vi "stiffbackReference.vi"() -> ()   [LabVIEW 2015]
uses:
  GlobalPath.vi
  GlobalData.vi
panel:
  in  "DONE ALL?":bool
  out "Mapping file Ext dx":string
  out "Mapping file Ext sx":string
  out "Mapping file Int dx":string
  out "Mapping file Int sx":string
  out "appended path":path
  out "Mapping file pillar":string
  in  "Open Program 5":bool
  out "PanelName":string
  in  "Done with reference plate mapping?":bool
  in  "Open Program":bool
  # "1. Stiffback plate mapping"
  # "At this point, the PCB on the table/stiffback will be tested in the appropriate vi program"
  # "PCB MAPPING"
  # "FRAME/COOLING BAR MAPPING"
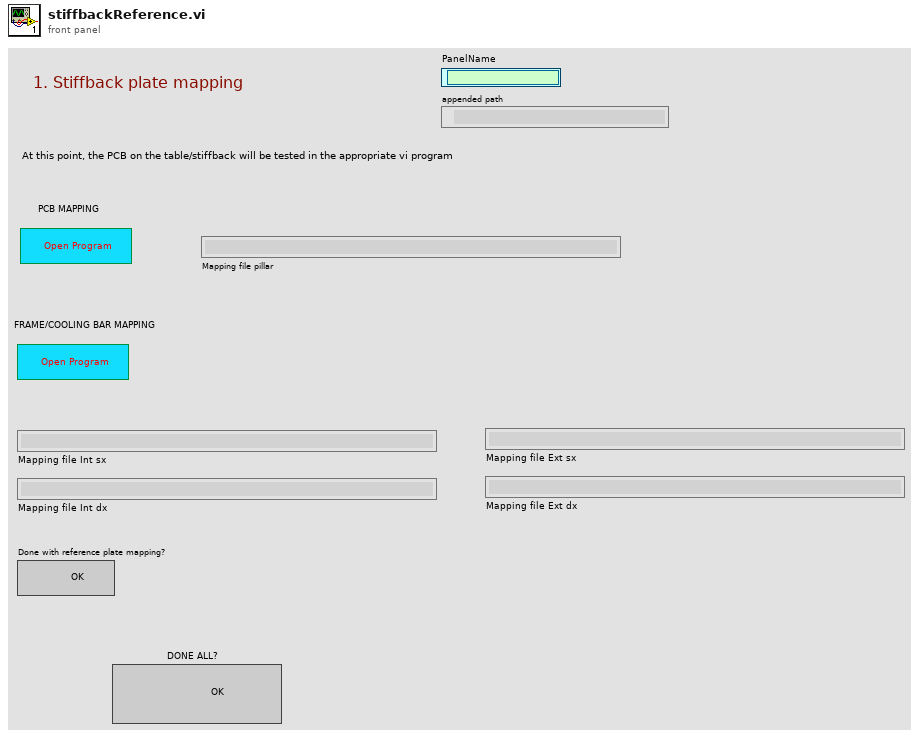
[diagram p1: front panel]
types:
  T1 = enum16{"open", "replace", "create", "open or create", "replace or create", "replace or create with confirmation"}
  T2 = enum32{"Bad", "Idle", "Run top level", "Running"}
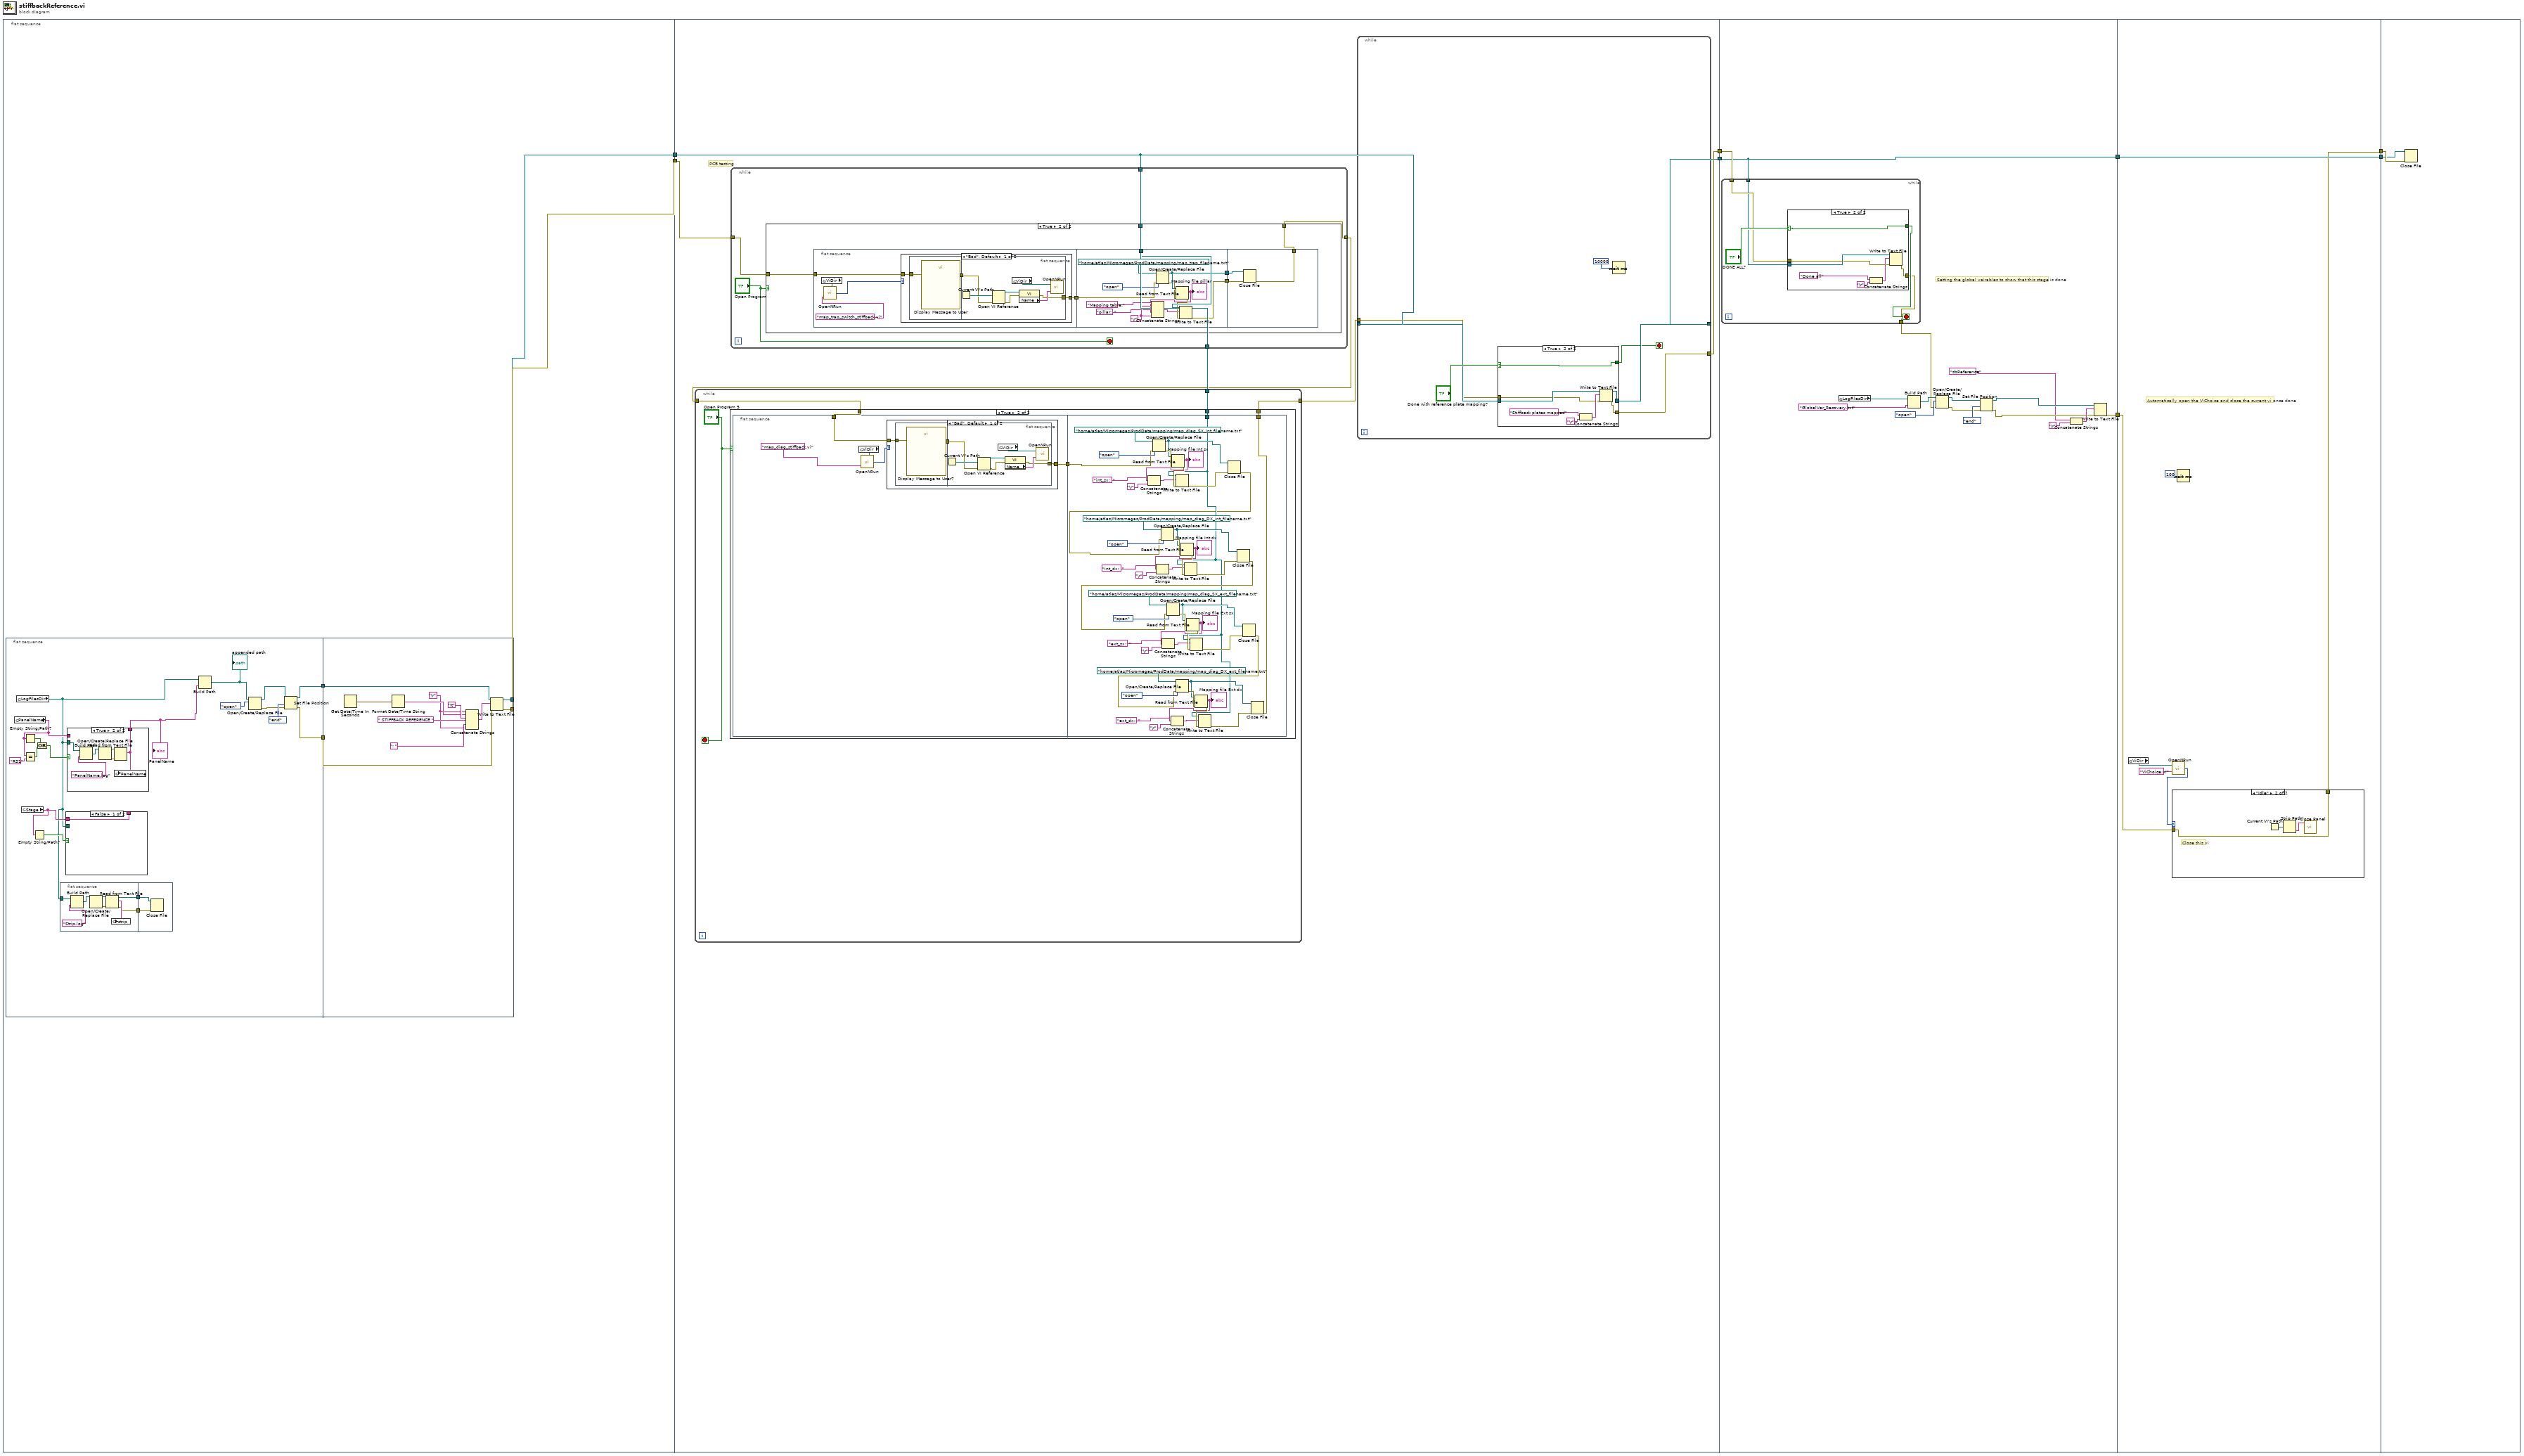
[diagram p0: block diagram]
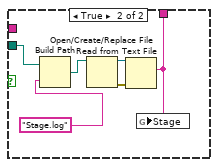
[diagram p2: hidden frame]
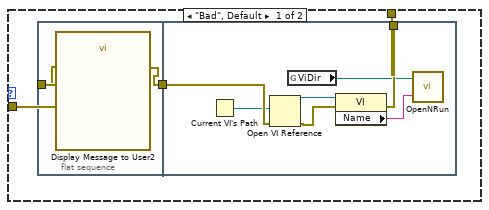
[diagram p10: hidden frame]
diagram:
  n1 = flat-sequence {
    tunnel: [w11] -> w2
    tunnel: [w9] -> w1
    tunnel: w2 -> [w72]
    tunnel: [w66] -> w8
    tunnel: [w71] -> w7
    tunnel: w1 -> [w67]
    tunnel: w8 -> [w212]
    tunnel: w7 -> [w210]
    tunnel: [w210] -> w6
    tunnel: [w214] -> w4
    tunnel: w6 -> [w245]
    tunnel: [w245] -> w5
    tunnel: w4 -> [w241]
    tunnel: [w240] -> w3
    tunnel: w5 -> [w261]
    tunnel: w3 -> [w262]
    frame #0 {
      n2 = flat-sequence {
        tunnel: [w25] -> w12
        tunnel: [w24] -> w10
        tunnel: w12 -> [w61]
        tunnel: [w60] -> w9
        tunnel: [w59] -> w11
        tunnel: w10 -> [w58]
        frame #0 {
          n3 = global read "GlobalData.vi" "PanelName"() -> (w18:string)
          n4 = global read "GlobalPath.vi" "LogFilesDir"() -> (w13:path)
          n5 = global read "GlobalData.vi" "Stage"() -> (w22:string)
          n6 = Empty String/Path?(string/path=w18) -> (empty?=w20:bool)
          n7 = Equal?(x=w18, y="RS1") -> (x = y?=w16:bool)
          n8 = Empty String/Path?(string/path=w22) -> (empty?=w23:bool)
          n9 = Or(x=w20, y=w16) -> (x .or. y?=w19:bool)
          n10 = flat-sequence {
            tunnel: w13 -> [w38]
            tunnel: [w32] -> w15
            tunnel: [w31] -> w14
            tunnel: w15 -> [w40]
            tunnel: w14 -> [w39]
            frame #0 {
              n11 = Build Path(base path=w38, name or relative path="Strip.log") -> (appended path=w37:path)
              n12 = Open/Create/Replace File(file path (use dialog)=w37) -> (refnum out=w34:refnum<file>, error out=w35:errorcluster)  [unwired: 5 in, 1 out]
              n13 = Read from Text File(file (use dialog)=w34, error in=w35) -> (refnum out=w31:refnum<file>, text=w33:string, error out=w32:errorcluster)  [unwired: 2 in, 1 out]
              n14 = global write "GlobalData.vi" "strip"(w33) -> ()
            }
            frame #1 {
              n15 = Close File(refnum=w39, error in=w40) -> ()  [unwired: 2 out]
            }
          }
          n16 = case shown="False" w23 {
            tunnel: w13 -> [_ w47]
            tunnel: [w41 w42] -> _
            tunnel: w22 -> [w41 _]
            frame False {
            }
            frame True {
              n17 = Build Path(base path=w47, name or relative path="Stage.log") -> (appended path=w46:path)
              n18 = Open/Create/Replace File(file path (use dialog)=w46) -> (refnum out=w43:refnum<file>, error out=w44:errorcluster)  [unwired: 5 in, 1 out]
              n19 = Read from Text File(file (use dialog)=w43, error in=w44) -> (text=w42:string)  [unwired: 2 in, 3 out]
              n20 = global write "GlobalData.vi" "Stage"(w42) -> ()
            }
          }
          n21 = case shown="True" w19 {
            tunnel: w13 -> [_ w54]
            tunnel: [w48 w49] -> w21
            tunnel: w18 -> [w48 _]
            frame False {
            }
            frame True {
              n22 = Build Path(base path=w54, name or relative path="PanelName.log") -> (appended path=w53:path)
              n23 = Open/Create/Replace File(file path (use dialog)=w53) -> (refnum out=w50:refnum<file>, error out=w51:errorcluster)  [unwired: 5 in, 1 out]
              n24 = Read from Text File(file (use dialog)=w50, error in=w51) -> (text=w49:string)  [unwired: 2 in, 3 out]
              n25 = global write "GlobalData.vi" "PanelName"(w49) -> ()
            }
          }
          "PanelName" <- w21
          n26 = Build Path(base path=w13, name or relative path=w21) -> (appended path=w30:path)
          "appended path" <- w30
          n27 = Open/Create/Replace File(file path (use dialog)=w30, operation (0:open)=T1."open") -> (refnum out=w27:refnum<file>, error out=w26:errorcluster)  [unwired: 4 in, 1 out]
          n28 = Set File Position(refnum=w27, from (0:start)=enum16{"start", "end", "current"}."end", error in=w26) -> (refnum out=w25:refnum<file>, error out=w24:errorcluster)  [unwired: 1 in]
        }
        frame #1 {
          w55 = "\r"
          n29 = Get Date/Time In Seconds() -> (seconds since 1Jan1904=w57:timestamp)
          n30 = Format Date/Time String(seconds (now)=w57) -> (date/time string=w63:string)  [unwired: 2 in]
          n31 = Concatenate Strings(w55, w63, "\t", " STIFFBACK REFERENCE ", ": ", w55) -> (w62:string)
          n32 = Write to Text File(file (use dialog)=w61, text=w62, error in=w58) -> (refnum out=w60:refnum<file>, error out=w59:errorcluster)  [unwired: 1 in, 1 out]
        }
      }
    }
    frame #1 {
      # "PCB testing"
      n33 = while {
        tunnel: w67 -> [w146]
        tunnel: [w146] -> w69
        tunnel: w72 -> [w148]
        tunnel: [w149] -> w68
        stop <- "Open Program" stop-if-true
        n34 = case shown="True" "Open Program" {
          tunnel: [w150 w155] -> w149
          tunnel: w148 -> [w150 w156]
          tunnel: w146 -> [_ w154]
          frame False {
          }
          frame True {
            n35 = flat-sequence {
              tunnel: w156 -> [w158]
              tunnel: [w157] -> w153
              tunnel: [w185] -> w152
              tunnel: [w180] -> w151
              tunnel: w153 -> [w183]
              tunnel: w154 -> [w182]
              tunnel: w152 -> [w190]
              tunnel: w151 -> [w189]
              tunnel: [w188] -> w155
              frame #0 {
                n36 = global read "GlobalPath.vi" "ViDir"() -> (w161:path)
                n37 = call "OpenNRun.vi"("VI name"="map_trap_switch_stiffback.vi", "ViDirPath"=w161) -> ("Execution:State"=w160:T2)
                n38 = case shown="\"Bad\", Default" w160 {
                  tunnel: [w164 w174] -> w157
                  tunnel: w158 -> [w163 w174]
                  frame "Bad", Default {
                    n39 = flat-sequence {
                      tunnel: w163 -> [w166]
                      tunnel: [w165] -> w162
                      tunnel: [w169] -> w164
                      tunnel: w162 -> [w167]
                      frame #0 {
                        n40 = call "Display Message to User"("error in (no error)"=w166) -> ("error out"=w165:errorcluster)  [unwired: 9 in, 1 out]
                      }
                      frame #1 {
                        n41 = Current VI's Path() -> (path=w168:path)
                        n42 = Open VI Reference(vi path=w168, error in (no error)=w167) -> (vi reference=w173:refnum<vi>, error out=w172:errorcluster)  [unwired: 4 in]
                        n43 = global read "GlobalPath.vi" "ViDir"() -> (w171:path)
                        n44 = property class="VI"(reference=w173, error in=w172) -> (error out=w169:errorcluster, "Name"=w170:string)  [unwired: 1 out]
                        n45 = call "OpenNRun.vi"("VI name"=w170, "ViDirPath"=w171) -> ()  [unwired: 1 out]
                      }
                    }
                  }
                  frame "Idle" {
                  }
                }
              }
              frame #1 {
                w177 = "\r"
                n46 = Open/Create/Replace File(file path (use dialog)=path "/home/atlas/Micromegas/ProdData/mapping/map_trap_filename.txt", error in=w183, operation (0:open)=T1."open") -> (refnum out=w185:refnum<file>, error out=w184:errorcluster)  [unwired: 3 in, 1 out]
                n47 = Read from Text File(file (use dialog)=w185, error in=w184) -> (text=w176:string, error out=w181:errorcluster)  [unwired: 2 in, 2 out]
                "Mapping file pillar" <- w176
                n48 = Concatenate Strings("Mapping table:", w177, "pillar:  ", w176, w177) -> (w179:string)
                n49 = Write to Text File(file (use dialog)=w182, text=w179, error in=w181) -> (error out=w180:errorcluster)  [unwired: 1 in, 2 out]
              }
              frame #2 {
                n50 = Close File(refnum=w190, error in=w189) -> (error out=w188:errorcluster)  [unwired: 1 out]
              }
            }
          }
        }
      }
      n51 = while {
        tunnel: w69 -> [w74]
        tunnel: w68 -> [w76]
        tunnel: [w73] -> w70
        stop <- "Open Program 5" stop-if-true
        n52 = case shown="True" "Open Program 5" {
          tunnel: w76 -> [w77 w81]
          tunnel: w74 -> [_ w79]
          tunnel: [w77 w78] -> w73
          frame False {
          }
          frame True {
            n53 = flat-sequence {
              tunnel: w81 -> [w84]
              tunnel: [w82] -> w80
              tunnel: w80 -> [w137]
              tunnel: w79 -> [w103]
              tunnel: [w100] -> w78
              frame #0 {
                n54 = global read "GlobalPath.vi" "ViDir"() -> (w86:path)
                n55 = call "OpenNRun.vi"("VI name"="map_diag_stiffback.vi", "ViDirPath"=w86) -> ("Execution:State"=w85:T2)
                n56 = case shown="\"Bad\", Default" w85 {
                  tunnel: [w89 w99] -> w82
                  tunnel: w84 -> [w88 w99]
                  frame "Bad", Default {
                    n57 = flat-sequence {
                      tunnel: w88 -> [w91]
                      tunnel: [w90] -> w87
                      tunnel: [w94] -> w89
                      tunnel: w87 -> [w92]
                      frame #0 {
                        n58 = call "Display Message to User7"("error in (no error)"=w91) -> ("error out"=w90:errorcluster)  [unwired: 9 in, 1 out]
                      }
                      frame #1 {
                        n59 = Current VI's Path() -> (path=w93:path)
                        n60 = Open VI Reference(vi path=w93, error in (no error)=w92) -> (vi reference=w98:refnum<vi>, error out=w97:errorcluster)  [unwired: 4 in]
                        n61 = global read "GlobalPath.vi" "ViDir"() -> (w96:path)
                        n62 = property class="VI"(reference=w98, error in=w97) -> (error out=w94:errorcluster, "Name"=w95:string)  [unwired: 1 out]
                        n63 = call "OpenNRun.vi"("VI name"=w95, "ViDirPath"=w96) -> ()  [unwired: 1 out]
                      }
                    }
                  }
                  frame "Idle" {
                  }
                }
              }
              frame #1 {
                n64 = Open/Create/Replace File(file path (use dialog)=path "/home/atlas/Micromegas/ProdData/mapping/map_diag_SX_int_filename.txt", error in=w137, operation (0:open)=T1."open") -> (refnum out=w135:refnum<file>, error out=w143:errorcluster)  [unwired: 3 in, 1 out]
                n65 = Read from Text File(file (use dialog)=w135, error in=w143) -> (text=w139:string, error out=w142:errorcluster)  [unwired: 2 in, 2 out]
                "Mapping file Int sx" <- w139
                n66 = Concatenate Strings("int_sx:  ", w139, "\r") -> (w141:string)
                n67 = Write to Text File(file (use dialog)=w103, text=w141, error in=w142) -> (error out=w136:errorcluster)  [unwired: 1 in, 2 out]
                n68 = Close File(refnum=w135, error in=w136) -> (error out=w101:errorcluster)  [unwired: 1 out]
                n69 = Open/Create/Replace File(file path (use dialog)=path "/home/atlas/Micromegas/ProdData/mapping/map_diag_DX_int_filename.txt", error in=w101, operation (0:open)=T1."open") -> (refnum out=w125:refnum<file>, error out=w132:errorcluster)  [unwired: 3 in, 1 out]
                n70 = Read from Text File(file (use dialog)=w125, error in=w132) -> (text=w128:string, error out=w131:errorcluster)  [unwired: 2 in, 2 out]
                "Mapping file Int dx" <- w128
                n71 = Concatenate Strings("int_dx:  ", w128, "\r") -> (w130:string)
                n72 = Write to Text File(file (use dialog)=w103, text=w130, error in=w131) -> (error out=w126:errorcluster)  [unwired: 1 in, 2 out]
                n73 = Close File(refnum=w125, error in=w126) -> (error out=w114:errorcluster)  [unwired: 1 out]
                n74 = Open/Create/Replace File(file path (use dialog)=path "/home/atlas/Micromegas/ProdData/mapping/map_diag_SX_ext_filename.txt", error in=w114, operation (0:open)=T1."open") -> (refnum out=w115:refnum<file>, error out=w122:errorcluster)  [unwired: 3 in, 1 out]
                n75 = Read from Text File(file (use dialog)=w115, error in=w122) -> (text=w118:string, error out=w121:errorcluster)  [unwired: 2 in, 2 out]
                "Mapping file Ext sx" <- w118
                n76 = Concatenate Strings("ext_sx:  ", w118, "\r") -> (w120:string)
                n77 = Write to Text File(file (use dialog)=w103, text=w120, error in=w121) -> (error out=w116:errorcluster)  [unwired: 1 in, 2 out]
                n78 = Close File(refnum=w115, error in=w116) -> (error out=w102:errorcluster)  [unwired: 1 out]
                n79 = Open/Create/Replace File(file path (use dialog)=path "/home/atlas/Micromegas/ProdData/mapping/map_diag_DX_ext_filename.txt", error in=w102, operation (0:open)=T1."open") -> (refnum out=w104:refnum<file>, error out=w111:errorcluster)  [unwired: 3 in, 1 out]
                n80 = Read from Text File(file (use dialog)=w104, error in=w111) -> (text=w107:string, error out=w110:errorcluster)  [unwired: 2 in, 2 out]
                "Mapping file Ext dx" <- w107
                n81 = Concatenate Strings("ext_dx:  ", w107, "\r") -> (w109:string)
                n82 = Write to Text File(file (use dialog)=w103, text=w109, error in=w110) -> (error out=w105:errorcluster)  [unwired: 1 in, 2 out]
                n83 = Close File(refnum=w104, error in=w105) -> (error out=w100:errorcluster)  [unwired: 1 out]
              }
            }
          }
        }
      }
      n84 = while {
        tunnel: w67 -> [w196]
        tunnel: w70 -> [w195]
        tunnel: [w194] -> w71
        tunnel: [w191] -> w66
        stop <- w192 stop-if-true
        n85 = case shown="True" "Done with reference plate mapping?" {
          selector: "Done with reference plate mapping?" -> [w200 w205]
          tunnel: [w200 w205] -> w192
          tunnel: w196 -> [w198 w204]
          tunnel: w195 -> [w199 w203]
          tunnel: [w199 w201] -> w191
          tunnel: [w198 w202] -> w194
          frame False {
          }
          frame True {
            n86 = Concatenate Strings("Stiffback plates mapped", "\r") -> (w208:string)
            n87 = Write to Text File(file (use dialog)=w204, text=w208, error in=w203) -> (refnum out=w202:refnum<file>, error out=w201:errorcluster)  [unwired: 1 in, 1 out]
          }
        }
        n88 = Wait (ms)(milliseconds to wait=10000) -> ()  [unwired: 1 out]
      }
    }
    frame #2 {
      # "Setting the global vairables to show that this stage is done"
      n89 = while {
        tunnel: w212 -> [w228]
        tunnel: [w225] -> w211
        tunnel: w210 -> [w227]
        stop <- w226 stop-if-true
        n90 = case shown="True" "DONE ALL?" {
          selector: "DONE ALL?" -> [w231 w232]
          tunnel: [w231 w232] -> w226
          tunnel: w227 -> [_ w235]
          tunnel: w228 -> [w230 w234]
          tunnel: [w230 w233] -> w225
          frame False {
          }
          frame True {
            n91 = Concatenate Strings("Done all", "\r") -> (w238:string)
            n92 = Write to Text File(file (use dialog)=w235, text=w238, error in=w234) -> (error out=w233:errorcluster)  [unwired: 1 in, 2 out]
          }
        }
      }
      n93 = global read "GlobalPath.vi" "LogFilesDir"() -> (w213:path)
      n94 = Build Path(base path=w213, name or relative path="GlobalVar_Recovery.txt") -> (appended path=w223:path)
      n95 = Open/Create/Replace File(file path (use dialog)=w223, error in=w211, operation (0:open)=T1."open") -> (refnum out=w219:refnum<file>, error out=w220:errorcluster)  [unwired: 3 in, 1 out]
      n96 = Set File Position(refnum=w219, from (0:start)=enum16{"start", "end", "current"}."end", error in=w220) -> (refnum out=w216:refnum<file>, error out=w215:errorcluster)  [unwired: 1 in]
      n97 = Concatenate Strings("sbReference", "\r") -> (w218:string)
      n98 = Write to Text File(file (use dialog)=w216, text=w218, error in=w215) -> (error out=w214:errorcluster)  [unwired: 1 in, 2 out]
    }
    frame #3 {
      # "Automatically open the ViChoice and close the current vi once done"
      n99 = global read "GlobalPath.vi" "ViDir"() -> (w244:path)
      n100 = call "OpenNRun.vi"("VI name"="ViChoice.vi", "ViDirPath"=w244) -> ("Execution:State"=w243:T2)
      n101 = case shown="\"Idle\"" w243 {
        tunnel: [w248 w258] -> w240
        tunnel: w241 -> [w246 w258]
        frame "Bad", Default {
          n102 = flat-sequence {
            tunnel: w246 -> [w250]
            tunnel: [w249] -> w247
            tunnel: [w254] -> w248
            tunnel: w247 -> [w253]
            frame #0 {
              n103 = call "Display Message to User2"("error in (no error)"=w250) -> ("error out"=w249:errorcluster)  [unwired: 9 in, 1 out]
            }
            frame #1 {
              n104 = Current VI's Path() -> (path=w251:path)
              n105 = Open VI Reference(vi path=w251, error in (no error)=w253) -> (vi reference=w257:refnum<vi>, error out=w256:errorcluster)  [unwired: 4 in]
              n106 = global read "GlobalPath.vi" "ViDir"() -> (w252:path)
              n107 = property class="VI"(reference=w257, error in=w256) -> (error out=w254:errorcluster, "Name"=w255:string)  [unwired: 1 out]
              n108 = call "OpenNRun.vi"("VI name"=w255, "ViDirPath"=w252) -> ()  [unwired: 1 out]
            }
          }
        }
        frame "Idle" {
          # "Close this vi"
          n109 = Current VI's Path() -> (path=w260:path)
          n110 = Strip Path(path=w260) -> (name=w259:string)  [unwired: 1 out]
          n111 = call <vilib>:"Close Panel.vi"("VI name"=w259) -> ()  [unwired: 10 in, 1 out]
        }
      }
      n112 = Wait (ms)(milliseconds to wait=100) -> ()  [unwired: 1 out]
    }
    frame #4 {
      n113 = Close File(refnum=w261, error in=w262) -> ()  [unwired: 2 out]
    }
  }
